vi "XY Graph Delete Successive Plots.vi"(8 "Error In":errorcluster, 9 "Plot Indices":i32[](array[numeric]), 11 "XYGraph Ref":refnum<vi>) -> (0 "Error Out":errorcluster, 1 "Plot Names":string[](array[string]), 2 "Graph Caption (or Label)":string, 3 "XYGraph Ref":refnum<vi>)   [LabVIEW 2019, in "XY Graph Add-Ons.lvlib"]
uses:
  XY Graph Add-Ons.lvlib
  Plot Update Steps.ctl
  XY Graph Plot Properties.ctl
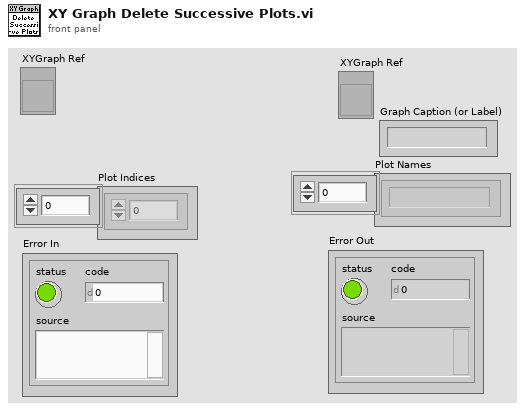
[diagram p1: front panel]
types:
  T1 = typedef "Plot Update Steps.ctl" = enum16{"Update Plot Styles", "Update Annotation List", "Update Cursor List", "Update Plots", "Quit"}
  T2 = typedef "XY Graph Plot Properties.ctl" = cluster{"Plot Index":i32, "Plot.Bar Plot Style":u8, "Plot.DigitalLineStyle":u8, "Plot.TransitionLocation":u8, "Plot.Transition Type":u8, "Plot.Fill To":i16, "Plot.Fill/Pt. Color":u32, "Plot.Label Format":u8, "Plot.Line Style":u8, "Plot.Line Width":u8, "Plot.Plot Color":u32, "Plot.Plot Interpolation":u8, "Plot.Plot Name":string, "Plot.Point Style":u8, "Plot.Visible?":bool, "Plot.XScaleIdx":u32, "Plot.YScaleIdx":u32, "Plot.Anti-aliased":bool}
  T3 = typedef "LVAnnotationListTypeDef.ctl" = cluster{"Name":string, "Color":u32, "Style":u8, "Point Style":u8, "Name Visible":bool, "Allow Drag":bool, "Annotation Mode":u32, "Plot":i32, "Index":i32, "Position":cluster{"X":dbl, "Y":dbl}, "X Scale":u32, "Y Scale":u32, "Show Arrow":bool, "Lock Name":bool, "Plot Area":i32, "Label Offset":cluster{"X":dbl, "Y":dbl}}[]
  T4 = typedef "LVCursorListTypeDef.ctl" = cluster{"Name":string, "Color":u32, "Style":u8, "Point Style":u8, "Name Visible":bool, "Allow Drag":bool, "Cursor Mode":u32, "Plot":i32, "Index":i32, "Position":cluster{"X":dbl, "Y":dbl}, "X Scale":u32, "Y Scale":u32, "Watch Plots":i32[], "Watch All Plots":bool, "Plot Area":i32, "Label Offset":cluster{"X":dbl, "Y":dbl}}[]
  T5 = typedef "XY Graph Add-Ons.lvlib/XY Graph Refnum.ctl" = refnum<vi>
  T6 = cluster{"Name":string, "Color":u32, "Style":u8, "Point Style":u8, "Name Visible":bool, "Allow Drag":bool, "Annotation Mode":u32, "Plot":i32, "Index":i32, "Position":cluster{"X":dbl, "Y":dbl}, "X Scale":u32, "Y Scale":u32, "Show Arrow":bool, "Lock Name":bool, "Plot Area":i32, "Label Offset":cluster{"X":dbl, "Y":dbl}}
  T7 = cluster{"Name":string, "Color":u32, "Style":u8, "Point Style":u8, "Name Visible":bool, "Allow Drag":bool, "Cursor Mode":u32, "Plot":i32, "Index":i32, "Position":cluster{"X":dbl, "Y":dbl}, "X Scale":u32, "Y Scale":u32, "Watch Plots":i32[], "Watch All Plots":bool, "Plot Area":i32, "Label Offset":cluster{"X":dbl, "Y":dbl}}
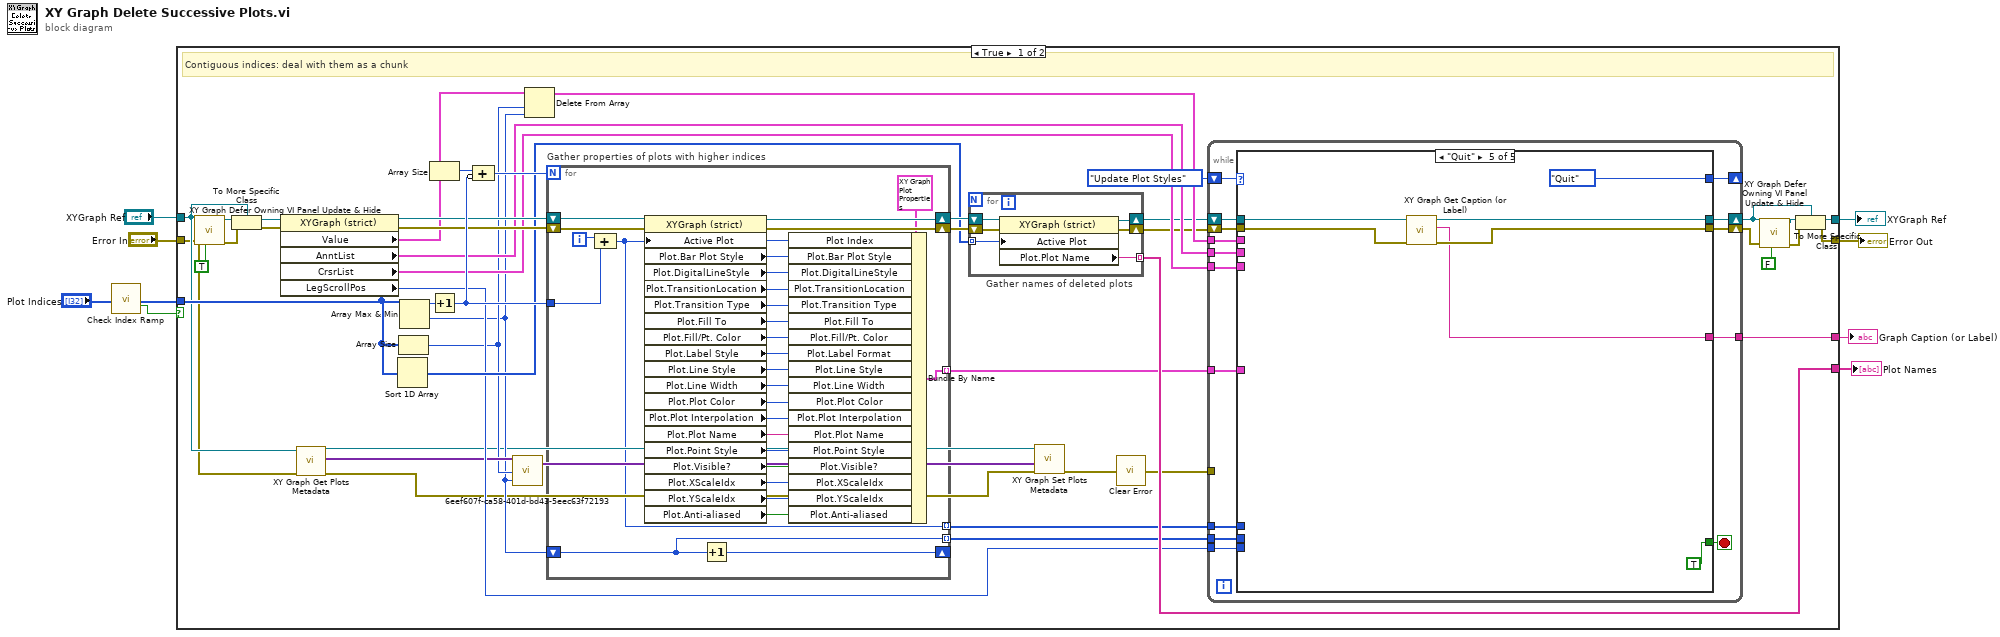
[diagram p0: block diagram]
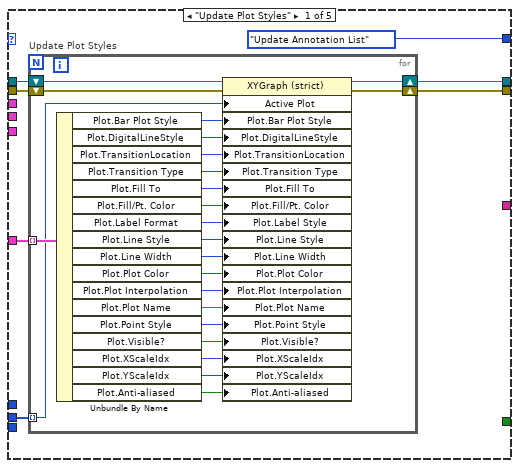
[diagram p2: hidden frame]
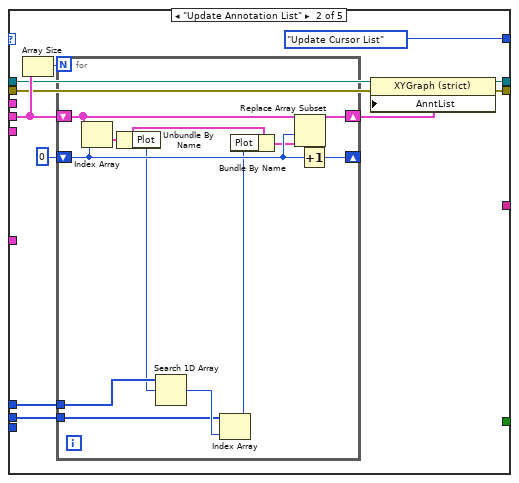
[diagram p3: hidden frame]
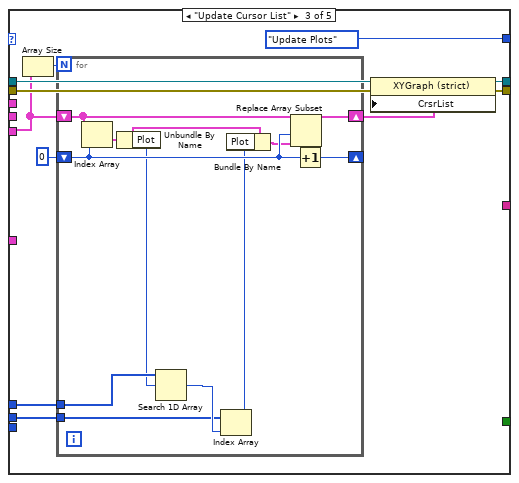
[diagram p4: hidden frame]
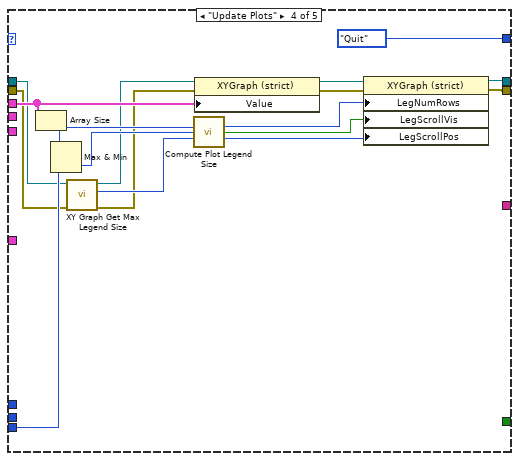
[diagram p5: hidden frame]
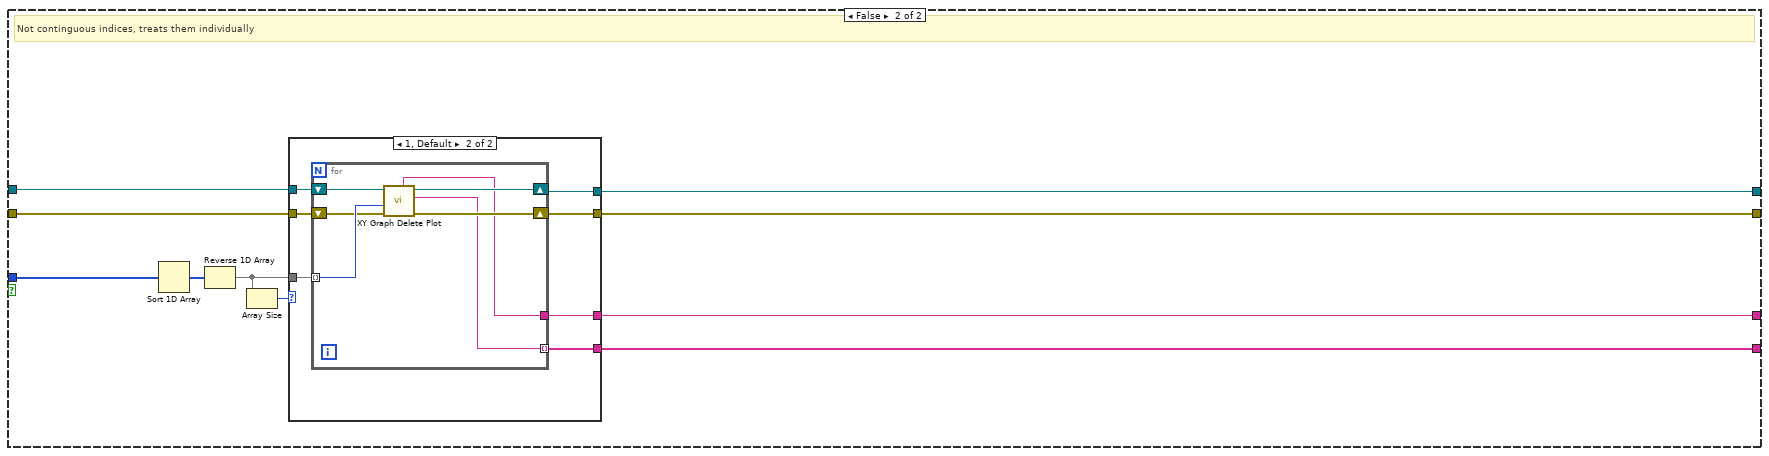
[diagram p6: hidden frame]
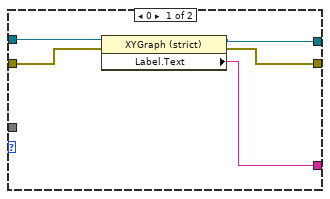
[diagram p7: hidden frame]
diagram:
  n1 = call "Check Index Ramp.vi"("Plot Indices"="Plot Indices") -> ("Plot Indices (dup)"=w1:i32[], "Contiguous?"=w2:bool)  [unwired: 16 in, 1 out]
  n2 = case shown="True" w2 {
    tunnel: "XYGraph Ref" -> [w19 w209]
    tunnel: [w23 w208] -> w8
    tunnel: "Error In" -> [w18 w207]
    tunnel: [w20 w206] -> w6
    tunnel: [w39 w205] -> w5
    tunnel: [w40 w204] -> w4
    tunnel: w1 -> [w46 w211]
    frame True {
      # "Contiguous indices: deal with them as a chunk"
      n3 = call "XY Graph Defer Owning VI Panel Update & Hide.vi"("Defer Owning Panel Update"=TRUE, "error in (no error)"=w18, "XY Graph Refnum in"=w19) -> ("error out"=w24:errorcluster, "XY Graph Refnum out"=w28:refnum<vi>)  [unwired: 7 in]
      n4 = To More Specific Class(target class=w19, reference=w28, error in=w24) -> (specific class reference=w26:refnum<vi>, error out=w25:errorcluster)
      n5 = property class="XYGraph (strict)"(reference=w26, error in=w25) -> (reference out=w49:refnum<vi>, error out=w48:errorcluster, "Value"=w47:cluster{dbl[], dbl[]}[], "AnntList"=w42:T3, "CrsrList"=w41:T4, "LegScrollPos"=w34:u32)
      n6 = call "XY Graph Get Plots Metadata.vi"("Error In"=w18, "XYGraph Ref"=w19) -> ("Error Out"=w14:errorcluster, "Plots Metadata"=w17:variant[], "XYGraph Ref (dup)"=w10:T5)  [unwired: 6 in, 1 out]
      n7 = Sort 1D Array(array=w46) -> (sorted array=w35:i32[])
      n8 = Array Size(array=w46) -> (size(s)=w16:i32)
      n9 = Array Max & Min(array=w46) -> (max value=w51:i32, min value=w15:i32)  [unwired: 2 out]
      n10 = Array Size(array=w47) -> (size(s)=w54:i32)
      n11 = Increment(x=w51) -> (x+1=w50:i32)
      n12 = Compound Arithmetic op=ADD(w54, invert w50) -> (w52:i32)
      n13 = call "6eef607f-ca58-401d-bd43-5eec63f72193.vi"("index (last elem)"=w15, "length (1)"=w16, "Array"=w17) -> ("array w/ subset deleted"=w11:variant[])  [unwired: 1 out]
      n14 = Delete From Array(array=w47, length=w16, index=w15) -> (array with subset deleted=w45:cluster{dbl[], dbl[]}[])  [unwired: 1 out]
      n15 = for "Gather properties of plots with higher indices" {
        N: w52 -> [_]
        shift-right: [w191] -> w43
        shift-left: w48 -> [w192]
        shift-right: [w193] -> w44
        shift-left: w49 -> [w195]
        tunnel: w50 -> [w173]
        shift-right: [w172] -> _
        shift-left: w15 -> [w171]
        tunnel: [w171] -> w38 mode=indexing
        tunnel: [w170] -> w37 mode=indexing
        tunnel: [w169] -> w36 mode=indexing
        i -> [w194]
        n16 = Compound Arithmetic op=ADD(w194, w173) -> (w169:i32)
        n17 = property class="XYGraph (strict)"(reference=w195, error in=w192, "Active Plot"=w169) -> (reference out=w193:refnum<vi>, error out=w191:errorcluster, "Plot.Bar Plot Style"=w190:u8, "Plot.DigitalLineStyle"=w189:u8, "Plot.TransitionLocation"=w188:u8, "Plot.Transition Type"=w187:u8, "Plot.Fill To"=w186:i16, "Plot.Fill/Pt. Color"=w185:u32, "Plot.Label Style"=w184:u8, "Plot.Line Style"=w183:u8, "Plot.Line Width"=w182:u8, "Plot.Plot Color"=w181:u32, "Plot.Plot Interpolation"=w180:u8, "Plot.Plot Name"=w179:string, "Plot.Point Style"=w178:u8, "Plot.Visible?"=w177:bool, "Plot.XScaleIdx"=w176:u32, "Plot.YScaleIdx"=w175:u32, "Plot.Anti-aliased"=w168:bool)
        n18 = Increment(x=w171) -> (x+1=w172:i32)
        n19 = Bundle By Name(cluster=T2 {"Plot Index"=0, "Plot.Bar Plot Style"=0, "Plot.DigitalLineStyle"=0, "Plot.TransitionLocation"=0, "Plot.Transition Type"=0, "Plot.Fill To"=0, "Plot.Fill/Pt. Color"=0, "Plot.Label Format"=0, "Plot.Line Style"=0, "Plot.Line Width"=0, "Plot.Plot Color"=0, "Plot.Plot Interpolation"=0, "Plot.Plot Name"="", "Plot.Point Style"=0, "Plot.Visible?"=FALSE, "Plot.XScaleIdx"=0, "Plot.YScaleIdx"=0, "Plot.Anti-aliased"=FALSE}, "Plot Index"=w169, "Plot.Bar Plot Style"=w190, "Plot.DigitalLineStyle"=w189, "Plot.TransitionLocation"=w188, "Plot.Transition Type"=w187, "Plot.Fill To"=w186, "Plot.Fill/Pt. Color"=w185, "Plot.Label Format"=w184, "Plot.Line Style"=w183, "Plot.Line Width"=w182, "Plot.Plot Color"=w181, "Plot.Plot Interpolation"=w180, "Plot.Plot Name"=w179, "Plot.Point Style"=w178, "Plot.Visible?"=w177, "Plot.XScaleIdx"=w176, "Plot.YScaleIdx"=w175, "Plot.Anti-aliased"=w168) -> (w170:T2)
      }
      n20 = for "Gather names of deleted plots" {
        shift-right: [w198] -> w32
        shift-left: w43 -> [w199]
        shift-right: [w200] -> w33
        shift-left: w44 -> [w201]
        tunnel: w35 -> [w197] mode=indexing
        tunnel: [w196] -> w40 mode=indexing
        n21 = property class="XYGraph (strict)"(reference=w201, error in=w199, "Active Plot"=w197) -> (reference out=w200:refnum<vi>, error out=w198:errorcluster, "Plot.Plot Name"=w196:string)
      }
      n22 = call "XY Graph Set Plots Metadata.vi"("error in (no error)"=w14, "Plots Metadata"=w11, "XY Graph Refnum"=w10) -> ("error out"=w13:errorcluster)  [unwired: 7 in, 1 out]
      n23 = call "Clear Error.vi"("Error In"=w13) -> ("no Error Out"=w12:errorcluster)  [unwired: 8 in]
      n24 = while {
        shift-right: [w64] -> _
        shift-left: Plot_Update_Steps."Update Plot Styles" -> [w66]
        shift-right: [w60] -> w31
        shift-left: w32 -> [w68]
        tunnel: w42 -> [w63]
        tunnel: w45 -> [w62]
        tunnel: w41 -> [w61]
        shift-right: [w67] -> w22
        shift-left: w33 -> [w69]
        tunnel: [w59] -> w39
        tunnel: w38 -> [w58]
        tunnel: w37 -> [w57]
        tunnel: w36 -> [w56]
        tunnel: w34 -> [w55]
        tunnel: w12 -> [_]
        stop <- w65 stop-if-true
        n25 = case shown="\"Quit\"" w66 {
          tunnel: w69 -> [w76 w106 w128 w146 w165]
          tunnel: w68 -> [w75 w104 w126 w147 w163]
          tunnel: [w74 w103 w125 w156 w162] -> w60
          tunnel: [w73 w105 w127 w157 w164] -> w67
          tunnel: w58 -> [w70 w101 w131 _ _]
          tunnel: [_ _ _ _ TRUE] -> w65
          tunnel: [Plot_Update_Steps."Update Annotation List" Plot_Update_Steps."Update Cursor List" Plot_Update_Steps."Update Plots" Plot_Update_Steps."Quit" Plot_Update_Steps."Quit"] -> w64
          tunnel: w63 -> [_ w109 _ _ _]
          tunnel: w62 -> [_ _ _ w159 _]
          tunnel: w61 -> [_ _ w123 _ _]
          tunnel: [_ _ _ _ w161] -> w59
          tunnel: w57 -> [w71 _ _ _ _]
          tunnel: w56 -> [_ w100 w122 _ _]
          tunnel: w55 -> [_ _ _ w153 _]
          frame "Update Plot Styles" {
            n26 = for "Update Plot Styles" {
              tunnel: w71 -> [w99] mode=indexing
              shift-right: [w95] -> w74
              shift-left: w75 -> [w96]
              shift-right: [w97] -> w73
              shift-left: w76 -> [w98]
              tunnel: w70 -> [w78] mode=indexing
              n27 = Unbundle By Name(w99) -> ("Plot.Bar Plot Style"=w94:u8, "Plot.DigitalLineStyle"=w93:u8, "Plot.TransitionLocation"=w92:u8, "Plot.Transition Type"=w91:u8, "Plot.Fill To"=w90:i16, "Plot.Fill/Pt. Color"=w89:u32, "Plot.Label Format"=w88:u8, "Plot.Line Style"=w87:u8, "Plot.Line Width"=w86:u8, "Plot.Plot Color"=w85:u32, "Plot.Plot Interpolation"=w84:u8, "Plot.Plot Name"=w83:string, "Plot.Point Style"=w82:u8, "Plot.Visible?"=w81:bool, "Plot.XScaleIdx"=w80:u32, "Plot.YScaleIdx"=w79:u32, "Plot.Anti-aliased"=w77:bool)
              n28 = property class="XYGraph (strict)"(reference=w98, error in=w96, "Active Plot"=w78, "Plot.Bar Plot Style"=w94, "Plot.DigitalLineStyle"=w93, "Plot.TransitionLocation"=w92, "Plot.Transition Type"=w91, "Plot.Fill To"=w90, "Plot.Fill/Pt. Color"=w89, "Plot.Label Style"=w88, "Plot.Line Style"=w87, "Plot.Line Width"=w86, "Plot.Plot Color"=w85, "Plot.Plot Interpolation"=w84, "Plot.Plot Name"=w83, "Plot.Point Style"=w82, "Plot.Visible?"=w81, "Plot.XScaleIdx"=w80, "Plot.YScaleIdx"=w79, "Plot.Anti-aliased"=w77) -> (reference out=w97:T5, error out=w95:errorcluster)
            }
          }
          frame "Update Annotation List" {
            n29 = Array Size(array=w109) -> (size(s)=w108:i32)
            n30 = for {
              N: w108 -> [_]
              shift-right: [w118] -> w102
              shift-left: w109 -> [w120]
              shift-right: [w117] -> _
              shift-left: 0 -> [w119]
              tunnel: w101 -> [w113]
              tunnel: w100 -> [w116]
              n31 = Index Array(array=w120, index=w119) -> (element=w121:T6)
              n32 = Unbundle By Name(w121) -> ("Plot"=w115:i32)
              n33 = Search 1D Array(1D array=w116, element=w115) -> (index of element=w114:i32)  [unwired: 1 in]
              n34 = Index Array(array=w113, index=w114) -> (element=w111:i32)
              n35 = Bundle By Name(cluster=w121, "Plot"=w111) -> (w112:T6)
              n36 = Replace Array Subset(array=w120, new element=w112, index=w119) -> (w118:T3)
              n37 = Increment(x=w119) -> (x+1=w117:i32)
            }
            n38 = property class="XYGraph (strict)"(reference=w106, error in=w104, "AnntList"=w102) -> (reference out=w105:T5, error out=w103:errorcluster)
          }
          frame "Update Cursor List" {
            n39 = Array Size(array=w123) -> (size(s)=w130:i32)
            n40 = for {
              N: w130 -> [_]
              tunnel: w131 -> [w135]
              shift-right: [w140] -> w124
              shift-left: w123 -> [w142]
              shift-right: [w139] -> _
              shift-left: 0 -> [w141]
              tunnel: w122 -> [w138]
              n41 = Index Array(array=w142, index=w141) -> (element=w143:T7)
              n42 = Unbundle By Name(w143) -> ("Plot"=w137:i32)
              n43 = Search 1D Array(1D array=w138, element=w137) -> (index of element=w136:i32)  [unwired: 1 in]
              n44 = Index Array(array=w135, index=w136) -> (element=w133:i32)
              n45 = Bundle By Name(cluster=w143, "Plot"=w133) -> (w134:T7)
              n46 = Replace Array Subset(array=w142, new element=w134, index=w141) -> (w140:T4)
              n47 = Increment(x=w141) -> (x+1=w139:i32)
            }
            n48 = property class="XYGraph (strict)"(reference=w128, error in=w126, "CrsrList"=w124) -> (reference out=w127:T5, error out=w125:errorcluster)
          }
          frame "Update Plots" {
            n49 = Array Size(array=w159) -> (size(s)=w154:i32)
            n50 = Max & Min(x=w154, y=w153) -> (min(x,y)=w152:u32)  [unwired: 1 out]
            n51 = call "XY Graph Get Max Legend Size.vi"("Error In"=w147, "XYGraph Refnum"=w146) -> ("Error Out"=w144:errorcluster, "Max Legend Size"=w148:i32, "XYGraph Refnum"=w145:T5)  [unwired: 6 in, 1 out]
            n52 = call "Compute Plot Legend Size.vi"("# Plots"=w154, "Current Plot (Last)"=w152, "Max Legend Size"=w148) -> ("LegNumRows"=w151:u32, "LegScrollVis"=w150:bool, "LegScrollPos"=w149:u32)  [unwired: 10 in]
            n53 = property class="XYGraph (strict)"(reference=w145, error in=w144, "Value"=w159) -> (reference out=w158:T5, error out=w155:errorcluster)
            n54 = property class="XYGraph (strict)"(reference=w158, error in=w155, "LegNumRows"=w151, "LegScrollVis"=w150, "LegScrollPos"=w149) -> (reference out=w157:T5, error out=w156:errorcluster)
          }
          frame "Quit" {
            n55 = call "XY Graph Get Caption (or Label).vi"("error in (no error)"=w163, "XYGraph in"=w165) -> ("error out"=w162:errorcluster, "Caption (or Label) Text"=w161:string, "XYGraph out"=w164:T5)  [unwired: 7 in]
          }
        }
      }
      n56 = call "XY Graph Defer Owning VI Panel Update & Hide.vi"("Defer Owning Panel Update"=FALSE, "error in (no error)"=w31, "XY Graph Refnum in"=w22) -> ("error out"=w21:errorcluster, "XY Graph Refnum out"=w30:refnum<vi>)  [unwired: 7 in]
      n57 = To More Specific Class(target class=w22, reference=w30, error in=w21) -> (specific class reference=w23:T5, error out=w20:errorcluster)
    }
    frame False {
      # "Not continguous indices, treats them individually"
      n58 = Sort 1D Array(array=w211) -> (sorted array=w210:i32[])
      n59 = Reverse 1D Array(array=w210) -> (reversed array=w203:i32[])
      n60 = Array Size(array=w203) -> (size(s)=w202:i32)
      n61 = case shown="1, Default" w202 {
        tunnel: w209 -> [w216 w223]
        tunnel: [w214 w222] -> w208
        tunnel: w207 -> [w215 w221]
        tunnel: [w213 w220] -> w206
        tunnel: [w212 w219] -> w205
        tunnel: [_ w218] -> w204
        tunnel: w203 -> [_ w217]
        frame 0 {
          n62 = property class="XYGraph (strict)"(reference=w216, error in=w215) -> (reference out=w214:refnum<vi>, error out=w213:errorcluster, "Label.Text"=w212:string)
        }
        frame 1, Default {
          n63 = for {
            tunnel: w217 -> [w229] mode=indexing
            shift-right: [w226] -> w220
            shift-left: w221 -> [w227]
            tunnel: [w225] -> w219
            tunnel: [w224] -> w218 mode=indexing
            shift-right: [w228] -> w222
            shift-left: w223 -> [w230]
            n64 = call "XY Graph Delete Plot.vi"("Error In"=w227, "Plot Index"=w229, "XYGraph Ref"=w230) -> ("Error Out"=w226:errorcluster, "Plot Name"=w224:string, "XYGraph Ref"=w228:T5, "Graph Caption (or Label)"=w225:string)  [unwired: 5 in]
          }
        }
      }
    }
  }
  "XYGraph Ref" <- w8
  "Error Out" <- w6
  "Graph Caption (or Label)" <- w5
  "Plot Names" <- w4
